vi "update.vi"(8 "error in (no error)":errorcluster, 11 "Context in":refnum<class "Context.lvclass">) -> (0 "error out":errorcluster, 3 "Context out":refnum<class "Context.lvclass">)   [LabVIEW 2013, in "Context.lvclass"]
uses:
  Context.lvclass
  Context.lvclass/Context.ctl
  State/State.lvclass
  Model/Model/Model.lvclass
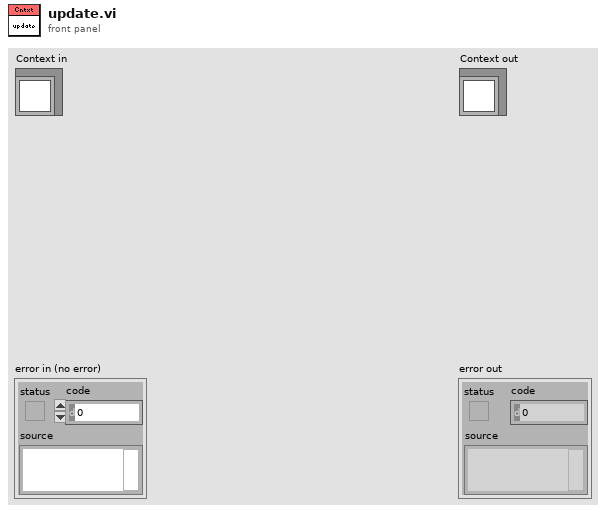
[diagram p1: front panel]
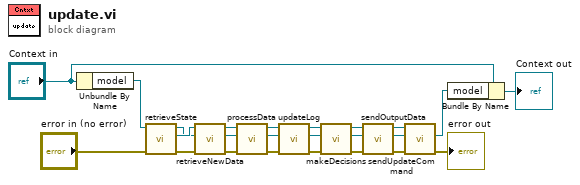
[diagram p0: block diagram]
diagram:
  n1 = Unbundle By Name("Context in") -> ("model"=w24:refnum<class "Model.lvclass">)
  n2 = call "retrieveState.vi"("error in (no error)"="error in (no error)", "Model in"=w24) -> ("error out"=w16:errorcluster, "state"=w20:refnum<class "State.lvclass">, "Model out"=w18:refnum<class "Model.lvclass">)  [unwired: 7 in]
  n3 = call-dynamic "retrieveNewData.vi"("error in (no error)"=w16, "model"=w18, "State in"=w20) -> ("error out"=w15:errorcluster, "model 2"=w17:refnum<class "Model.lvclass">, "State out"=w19:refnum<class "State.lvclass">)  [unwired: 6 in]
  n4 = call-dynamic "processData.vi"("error in (no error)"=w15, "model"=w17, "State in"=w19) -> ("error out"=w6:errorcluster, "model 2"=w7:refnum<class "Model.lvclass">, "State out"=w8:refnum<class "State.lvclass">)  [unwired: 6 in]
  n5 = call-dynamic "updateLog.vi"("error in (no error)"=w6, "model"=w7, "State in"=w8) -> ("error out"=w3:errorcluster, "model 2"=w4:refnum<class "Model.lvclass">, "State out"=w5:refnum<class "State.lvclass">)  [unwired: 6 in]
  n6 = call-dynamic "makeDecisions.vi"("error in (no error)"=w3, "model"=w4, "State in"=w5) -> ("error out"=w9:errorcluster, "model 2"=w10:refnum<class "Model.lvclass">, "State out"=w11:refnum<class "State.lvclass">)  [unwired: 6 in]
  n7 = call-dynamic "sendOutputData.vi"("error in (no error)"=w9, "model"=w10, "State in"=w11) -> ("error out"=w13:errorcluster, "model 2"=w12:refnum<class "Model.lvclass">, "State out"=w14:refnum<class "State.lvclass">)  [unwired: 6 in]
  n8 = call-dynamic "sendUpdateCommand.vi"("error in (no error)"=w13, "model"=w12, "State in"=w14) -> ("error out"=→"error out":errorcluster, "model 2"=w2:refnum<class "Model.lvclass">)  [unwired: 6 in, 1 out]
  n9 = Bundle By Name(cluster="Context in", "model"=w2) -> (→"Context out":refnum<class "Context.lvclass">)
